vi "proc_append_error.vi"(8 "error in":errorcluster, 11 "code in":i32) -> (0 "error out":errorcluster, 3 "code out":i32)   [LabVIEW 2011]
doc: "Appends LV process error text to error signal."
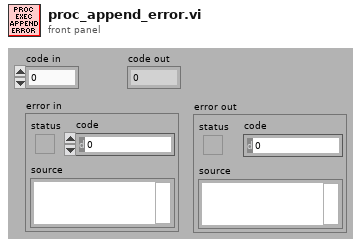
[diagram p1: front panel]
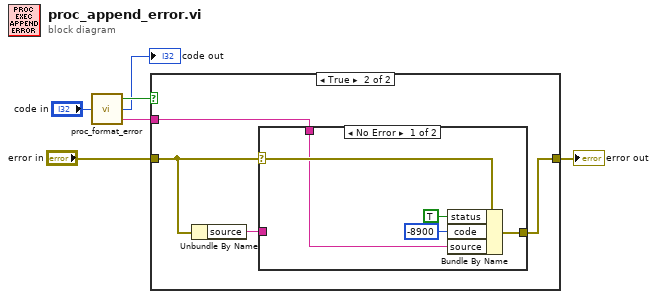
[diagram p0: block diagram]
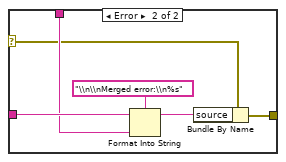
[diagram p3: hidden frame]
diagram:
  n1 = call "proc_format_error.vi"("code in"="code in") -> ("error"=w5:bool, "code out"=→"code out":i32, "error string"=w3:string)
  n2 = case shown="True" w5 {
    tunnel: "error in" -> [w7 w11]
    tunnel: w3 -> [_ w10]
    tunnel: [w7 w8] -> w2
    frame False {
    }
    frame True {
      n3 = Unbundle By Name(w11) -> ("source"=w9:string)
      n4 = case shown="No Error" w11 {
        selector: w11 -> [w16 w18]
        tunnel: w10 -> [w13 w20]
        tunnel: [w12 w17] -> w8
        tunnel: w9 -> [_ w22]
        frame No Error {
          n5 = Bundle By Name(cluster=w16, "status"=TRUE, "code"=-8900, "source"=w13) -> (w12:errorcluster)
        }
        frame Error {
          n6 = Format Into String(format string="\\n\\nMerged error:\\n%s", initial string=w22, w20) -> (resulting string=w19:string)  [unwired: 1 in, 1 out]
          n7 = Bundle By Name(cluster=w18, "source"=w19) -> (w17:errorcluster)
        }
      }
    }
  }
  "error out" <- w2
